vi "Post_AuthenticationCode_Request.vi"(8 "error in (no error)":errorcluster, 11 "OAuth in":refnum<class "OAuth.lvclass">) -> (0 "error out":errorcluster, 2 "Refresh Token":string, 3 "OAuth out":refnum<class "OAuth.lvclass">)   [LabVIEW 2016, in "OAuth.lvclass"]
uses:
  OAuth.lvclass
  OAuth.lvclass/OAuth.ctl
  <vilib>/httpClient/POSTBuffer.vi
  <vilib>/httpClient/LabVIEWHTTPClient.lvlib
  <vilib>/addons/_JKI.lib/Serialization/JSON/JKI JSON Serialization.lvlib
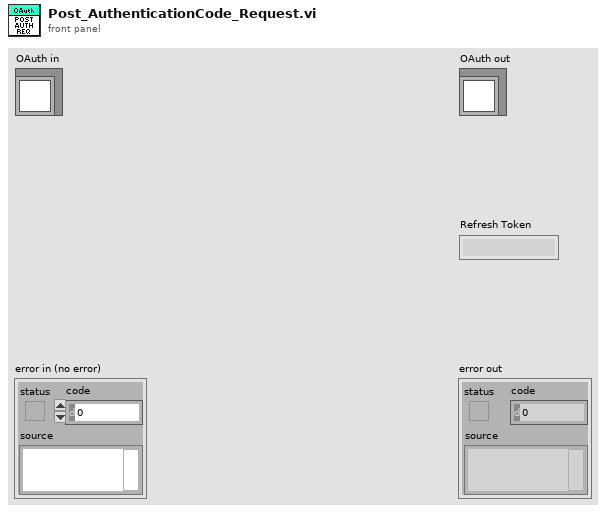
[diagram p1: front panel]
types:
  T1 = cluster{"token_type":string, "scope":string, "access_token":string, "refresh_token":string, "user_id":string, "expires_in":i32}
  T2 = typedef "LabVIEWHTTPClient.lvlib/ClientHandle.ctl" = refnum<k1>
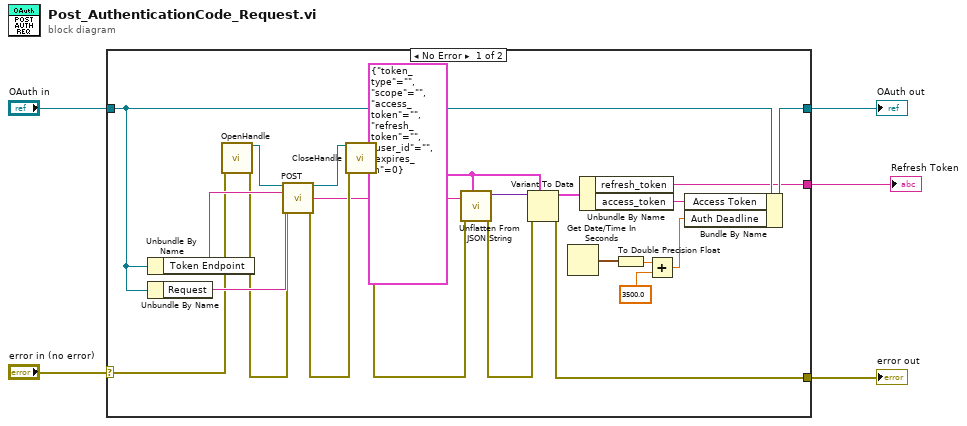
[diagram p0: block diagram]
diagram:
  n1 = case shown="No Error" "error in (no error)" {
    selector: "error in (no error)" -> [w10 w29]
    tunnel: [w9 w29] -> w4
    tunnel: [w12 w28] -> w2
    tunnel: "OAuth in" -> [w11 w28]
    tunnel: [w7 _] -> w1
    frame No Error {
      w21 = T1 {"token_type"="", "scope"="", "access_token"="", "refresh_token"="", "user_id"="", "expires_in"=0}
      n2 = Unbundle By Name(w11) -> ("Token Endpoint"=w25:string)
      n3 = Unbundle By Name(w11) -> ("Request"=w24:string)
      n4 = call <vilib>:"OpenHandle.vi"("error in (no error)"=w10) -> ("client handle out"=w27:T2, "error out"=w23:errorcluster)  [unwired: 13 in]
      n5 = call-poly <vilib>:"POST.vi"("client handle"=w27, "url"=w25, "buffer"=w24, "error in (no error)"=w23) -> ("client handle out"=w26:T2, "body"=w6:string, "error out"=w22:errorcluster)  [unwired: 8 in, 1 out]
      n6 = call <vilib>:"CloseHandle.vi"("client handle"=w26, "error in (no error)"=w22) -> ("error out"=w18:errorcluster)  [unwired: 13 in]
      n7 = call <vilib>:"Unflatten From JSON String.vi"("Type and Defaults"=w21, "error in (no error)"=w18, "JSON String"=w6) -> ("error out"=w17:errorcluster, "Variant"=w20:variant)  [unwired: 7 in]
      n8 = Variant To Data(error in=w17, type=w21, Variant=w20) -> (data=w19:T1, error out=w9:errorcluster)
      n9 = Get Date/Time In Seconds() -> (seconds since 1Jan1904=w14:timestamp)
      n10 = Unbundle By Name(w19) -> ("refresh_token"=w7:string, "access_token"=w8:string)
      n11 = To Double Precision Float(number=w14) -> (double precision float=w15:dbl)
      n12 = Add(x=w15, y=3500.0) -> (x+y=w13:dbl)
      n13 = Bundle By Name(cluster=w11, "Access Token"=w8, "Auth Deadline"=w13) -> (w12:refnum<class "OAuth.lvclass">)
    }
    frame Error {
    }
  }
  "error out" <- w4
  "OAuth out" <- w2
  "Refresh Token" <- w1
